vi "Take_next_trial.vi"(10 "Trial sequence in":cluster{"Sequence name":string, "Active":bool}[](array[cluster]), 11 "Remaining trials in":cluster{"Sequence name":string, "Active":bool}[](array[cluster])) -> (1 "Trial sequence out":cluster{"Sequence name":string, "Active":bool}[](array[cluster]), 2 "Remaining trials out":cluster{"Sequence name":string, "Active":bool}[](array[cluster]), 3 "Next trial":cluster{"Sequence name":string, "Active":bool})   [LabVIEW 2016]
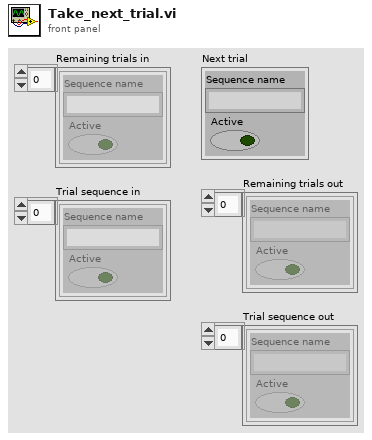
[diagram p1: front panel]
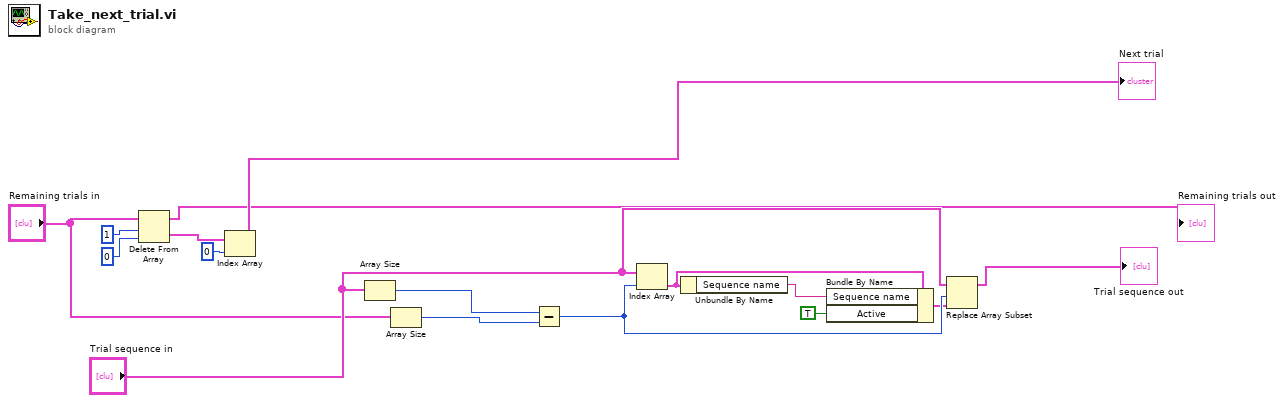
[diagram p0: block diagram]
diagram:
  n1 = Delete From Array(array="Remaining trials in", length=1, index=0) -> (deleted portion=w3:cluster{"Sequence name":string, "Active":bool}[], array with subset deleted=→"Remaining trials out":cluster{"Sequence name":string, "Active":bool}[])
  n2 = Index Array(array=w3, index=0) -> (element=→"Next trial":cluster{"Sequence name":string, "Active":bool})
  n3 = Array Size(array="Trial sequence in") -> (size(s)=w7:i32)
  n4 = Array Size(array="Remaining trials in") -> (size(s)=w9:i32)
  n5 = Subtract(x=w7, y=w9) -> (x-y=w14:i32)
  n6 = Index Array(array="Trial sequence in", index=w14) -> (element=w12:cluster{"Sequence name":string, "Active":bool})
  n7 = Unbundle By Name(w12) -> ("Sequence name"=w13:string)
  n8 = Bundle By Name(cluster=w12, "Sequence name"=w13, "Active"=TRUE) -> (w6:cluster{"Sequence name":string, "Active":bool})
  n9 = Replace Array Subset(array="Trial sequence in", new element=w6, index=w14) -> (→"Trial sequence out":cluster{"Sequence name":string, "Active":bool}[])
